vi "1B_Check JTAG Communication.vi"() -> ()   [LabVIEW 2010]
panel:
  out "Device Vcc":i32
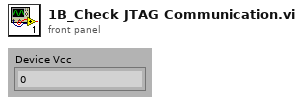
[diagram p1: front panel]
types:
  T1 = enum16{"--Disconnect All--", "Connect PulseGen to CH1", "Connect PulseGen to CH2", "Connect PulseGen to CH3", "Connect PulseGen to CH4", "Connect PulseGen to CH5", "Connect PulseGen to CH6", "Connect PulseGen to CH7", "Connect PulseGen to CH8", "Connect PulseGen to CH9", "Connect PulseGen to CH10", "Connect PulseGen to CH11", "Connect PulseGen to CH12", "Connect PulseGen to CH13", "Connect PulseGen to CH14", "Connect PulseGen to CH15", "Connect PulseGen to CH16", "Connect PulseGen to CH17", "Connect PulseGen to CH18", "Connect PulseGen to CH19", "Connect PulseGen to CH20", "Connect PulseGen to CH21", "Connect PulseGen to CH22", "Connect PulseGen to CH23", "Connect PulseGen to CH24", "Connect PulseGen to CH25", "Set MAG_SW", "Set Dynamic Load", "Set Expansion Trigger", "Trigger Positive Pulse", "Trigger Negative Pulse", "Set MSP Magic Pin", "Set BAT_EN", "Connect MSP_ACLK to CTR", "Connect MSP_MCLK to CTR", "Connect MSP_DIG_TST_OUT to CTR", "Connect STIM_SCK to CTR", "Connect STIM_CLK to CTR", "Connect SMU2 to Magnet", "Magnet Enable", "Cap Short", "Connect Positive Pulse to Pulse Bus", "Connect Negative Pulse to Pulse Bus", "Connect JTAG", "Connect JTAG DVDD Power", "RF Attach", "Connect SMU3 to VBAT", "Connect SMU3 Soft Start", "Connect ARB to Charge Coil", "Connect ARB to Matrix", "Connect CTR to Matrix", "DMM_I Short", "DMM_I 1000 Ohm", "DMM_I 100 Ohm", "DMM_I 10 Ohm", "Connect CH25 to DUT GND"}
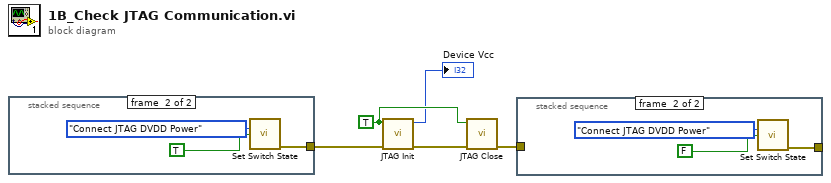
[diagram p0: block diagram]
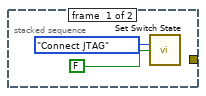
[diagram p2: hidden frame]
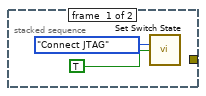
[diagram p3: hidden frame]
diagram:
  w3 = TRUE ("Power Target Device")
  n1 = stacked-sequence {
    tunnel: [_ w8] -> w5
    frame #0 {
      n2 = call "Set Switch State.vi"("Action"=T1."Connect JTAG", "State"=TRUE) -> ()  [unwired: 13 in, 1 out]
    }
    frame #1 {
      n3 = call "Set Switch State.vi"("Action"=T1."Connect JTAG DVDD Power", "State"=TRUE) -> ("error out"=w8:errorcluster)  [unwired: 13 in]
    }
  }
  n4 = call "JTAG Init.vi"("error in (no error)"=w5, "Power Target Device"=w3) -> ("error out"=w4:errorcluster, "Device Vcc"=→"Device Vcc":i32)  [unwired: 8 in]
  n5 = call "JTAG Close.vi"("error in (no error)"=w4, "Power Target Device"=w3) -> ("error out"=w2:errorcluster)  [unwired: 9 in]
  n6 = stacked-sequence {
    tunnel: [_ w13] -> _
    tunnel: w2 -> [_ _]
    frame #0 {
      n7 = call "Set Switch State.vi"("Action"=T1."Connect JTAG", "State"=FALSE) -> ()  [unwired: 13 in, 1 out]
    }
    frame #1 {
      n8 = call "Set Switch State.vi"("Action"=T1."Connect JTAG DVDD Power", "State"=FALSE) -> ("error out"=w13:errorcluster)  [unwired: 13 in]
    }
  }
